vi "And Operation (64).vi"(1 "X":bool[](array[boolean])=[FALSE, FALSE, FALSE, FALSE, FALSE, FALSE, FALSE, FALSE, FALSE, FALSE, FALSE, FALSE, FALSE, FALSE, FALSE, FALSE, FALSE, FALSE, FALSE, FALSE, FALSE, FALSE, FALSE, FALSE, FALSE, FALSE, FALSE, FALSE, FALSE, FALSE, FALSE, FALSE, FALSE, FALSE, FALSE, FALSE, FALSE, FALSE, FALSE, FALSE, FALSE, FALSE, FALSE, FALSE, FALSE, FALSE, FALSE, FALSE, FALSE, FALSE, FALSE, FALSE, FALSE, FALSE, FALSE, FALSE, FALSE, FALSE, FALSE, FALSE, FALSE, FALSE, FALSE, FALSE], 2 "Y":bool[](array[boolean])=[FALSE, FALSE, FALSE, FALSE, FALSE, FALSE, FALSE, FALSE, FALSE, FALSE, FALSE, FALSE, FALSE, FALSE, FALSE, FALSE, FALSE, FALSE, FALSE, FALSE, FALSE, FALSE, FALSE, FALSE, FALSE, FALSE, FALSE, FALSE, FALSE, FALSE, FALSE, FALSE, FALSE, FALSE, FALSE, FALSE, FALSE, FALSE, FALSE, FALSE, FALSE, FALSE, FALSE, FALSE, FALSE, FALSE, FALSE, FALSE, FALSE, FALSE, FALSE, FALSE, FALSE, FALSE, FALSE, FALSE, FALSE, FALSE, FALSE, FALSE, FALSE, FALSE, FALSE, FALSE]) -> (6 "X.and.Y?":bool[](array[boolean]))   [LabVIEW 2011]
doc: "This VI performs AND Operation on two 64 sized arrays"
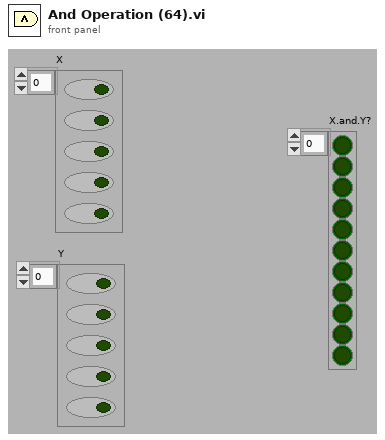
[diagram p1: front panel]
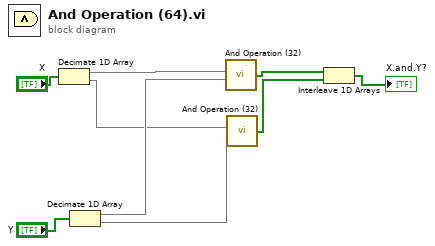
[diagram p0: block diagram]
diagram:
  n1 = Decimate 1D Array("X") -> (w7:bool[], w5:bool[])
  n2 = Decimate 1D Array("Y") -> (w6:bool[], w4:bool[])
  n3 = call <userlib>:"And Operation (32).vi"("X"=w7, "Y"=w6) -> ("X.and.Y?"=w2:bool[])  [unwired: 5 in]
  n4 = call <userlib>:"And Operation (32).vi"("X"=w5, "Y"=w4) -> ("X.and.Y?"=w3:bool[])  [unwired: 5 in]
  n5 = Interleave 1D Arrays(w2, w3) -> (→"X.and.Y?":bool[])
